vi "Create-message.vi"(8 "error in (no error)":errorcluster, 10 "Message type":T1) -> (0 "error out":errorcluster, 2 "Message out":refnum<class "Message.lvclass">)   [LabVIEW 2013, in "Server.lvlib" / "Server.lvclass"]
uses:
  Server.lvclass
  Messages/Sources/Message.lvclass
  Server-messages.ctl
  Messages/Sources/Heartbeat/Heartbeat.lvclass
  Messages/Sources/Get-clients/Get-clients.lvclass
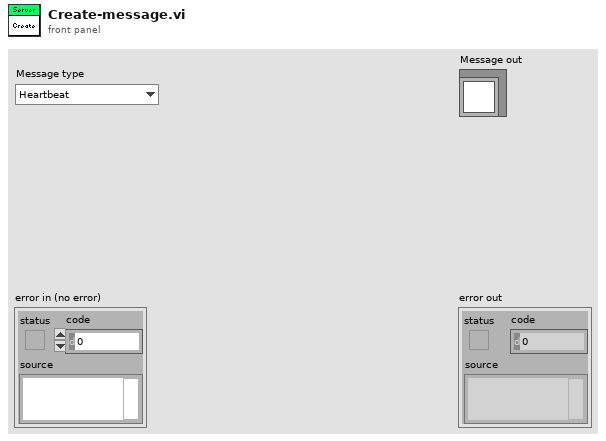
[diagram p1: front panel]
types:
  T1 = typedef "Server.lvlib/Server.lvclass/Server-messages.ctl" = enum16{"Heartbeat", "Error", "Start client", "Client stopped", "Query status", "Send status", "Get clients"}
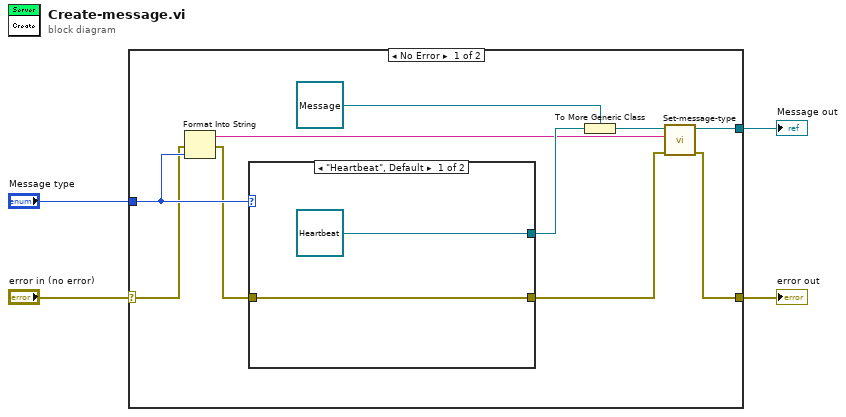
[diagram p0: block diagram]
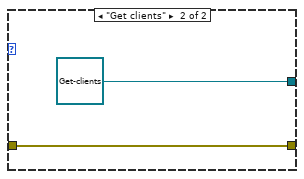
[diagram p2: hidden frame]
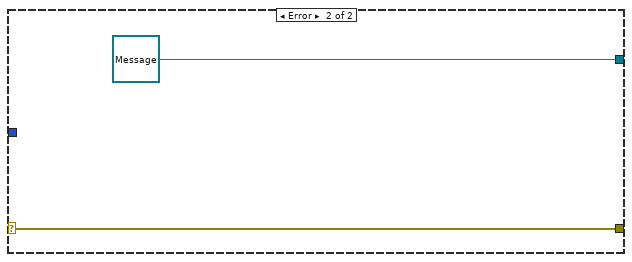
[diagram p3: hidden frame]
diagram:
  n1 = case shown="No Error" "error in (no error)" {
    selector: "error in (no error)" -> [w11 w20]
    tunnel: [w6 w20] -> w3
    tunnel: [w8 refnum<class "Message.lvclass"> refnum ("Module-communication.lvlib:Message.lvclass")] -> w2
    tunnel: "Message type" -> [w12 _]
    frame No Error {
      n2 = Format Into String(error in=w11, w12) -> (resulting string=w7:string, error out=w10:errorcluster)  [unwired: 2 in]
      n3 = case shown="\"Heartbeat\", Default" w12 {
        tunnel: w10 -> [w16 w18]
        tunnel: [w16 w18] -> w5
        tunnel: [refnum<class "Heartbeat.lvclass"> refnum ("Module-communication.lvlib:Heartbeat.lvclass") refnum<class "Get-clients.lvclass"> refnum ("Module-communication.lvlib:Get-clients.lvclass")] -> w14
        frame "Heartbeat", Default {
        }
        frame "Get clients" {
        }
      }
      n4 = To More Generic Class(target class=refnum<class "Message.lvclass"> refnum ("Module-communication.lvlib:Message.lvclass"), reference=w14) -> (generic class reference=w9:refnum<class "Message.lvclass">)
      n5 = call-dynamic "Set-message-type.vi"("error in (no error)"=w5, "Message type"=w7, "Message in"=w9) -> ("error out"=w6:errorcluster, "Message out"=w8:refnum<class "Message.lvclass">)  [unwired: 7 in]
    }
    frame Error {
    }
  }
  "error out" <- w3
  "Message out" <- w2
